vi "Replace Class Controls.vi"(8 "error in (no error)":errorcluster, 11 "Mock Class Generator In":refnum<class "Mock Class Generator.lvclass">) -> (0 "error out":errorcluster, 3 "Mock Class Generator Out":refnum<class "Mock Class Generator.lvclass">)   [LabVIEW 2020, in "Mock Class Generator.lvclass"]
uses:
  Mock Class Generator.lvclass
  Mock Class Generator.lvclass/Mock Class Generator.ctl
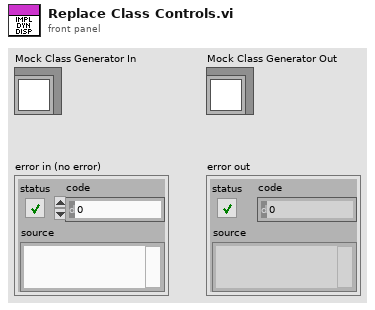
[diagram p1: front panel]
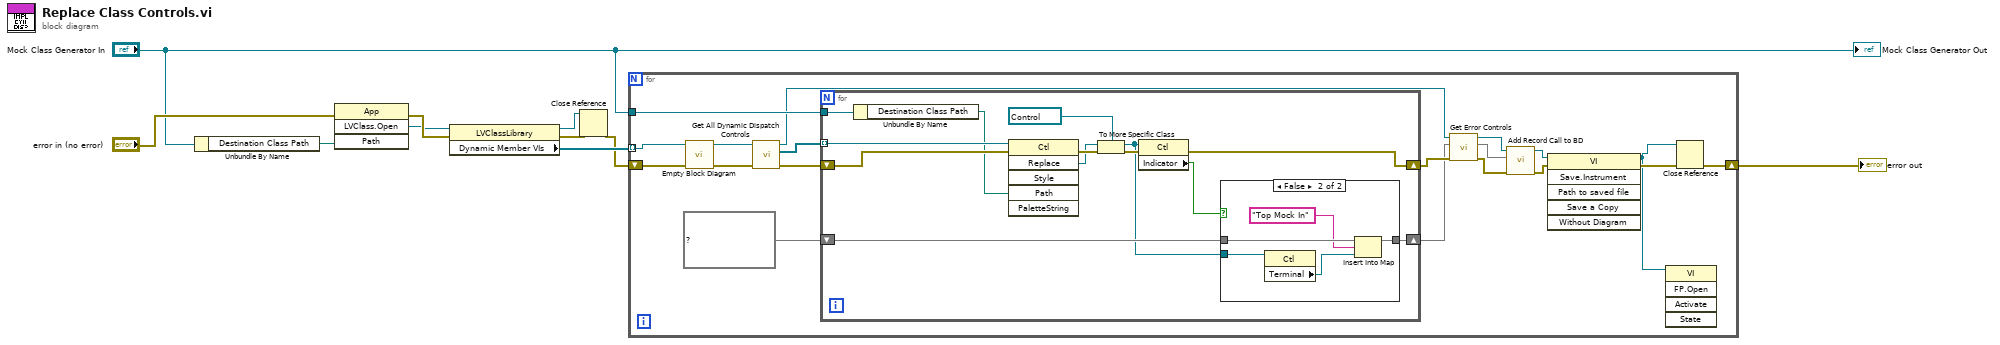
[diagram p0: block diagram]
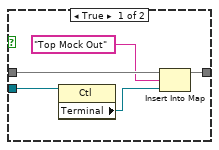
[diagram p2: hidden frame]
diagram:
  n1 = Unbundle By Name("Mock Class Generator In") -> ("Destination Class Path"=w10:path)
  n2 = invoke class="App" method="LVClass.Open"(error in="error in (no error)", "Path"=w10) -> (error out=w9:errorcluster, "LVClass.Open"=w4:refnum<vi>)  [unwired: 2 in, 2 out]
  n3 = property class="LVClassLibrary"(reference=w4, error in=w9) -> (reference out=w5:refnum<vi>, error out=w6:errorcluster, "Dynamic Member VIs"=w7:refnum<vi>[])
  n4 = Close Reference(reference=w5, error in (no error)=w6) -> (error out=w3:errorcluster)
  n5 = for {
    tunnel: w7 -> [w24] mode=indexing
    tunnel: "Mock Class Generator In" -> [w28]
    shift-right: [w25] -> w1
    shift-left: w3 -> [w21]
    n6 = call "Empty Block Diagram.vi"("error in (no error)"=w21, "VI in"=w24) -> ("error out"=w22:errorcluster, "reference out"=w23:refnum<vi>)  [unwired: 8 in]
    n7 = call "Get All Dynamic Dispatch Controls.vi"("error in (no error)"=w22, "VI in"=w23) -> ("error out"=w29:errorcluster, "Dynamic Dispatch Controls"=w27:refnum<vi>[], "reference out"=w19:refnum<vi>)  [unwired: 7 in]
    n8 = for {
      tunnel: w27 -> [w42] mode=indexing
      shift-right: [w34] -> w20
      shift-left: w29 -> [w41]
      tunnel: w28 -> [w40]
      shift-right: [w32] -> w13
      shift-left: map{string, refnum<vi>} {} ("map") -> [w33]
      n9 = Unbundle By Name(w40) -> ("Destination Class Path"=w39:path)
      n10 = invoke class="Ctl" method="Replace"(reference=w42, error in=w41, "Path"=w39) -> (error out=w38:errorcluster, "Replace"=w36:refnum<vi>)  [unwired: 3 in, 4 out]
      n11 = To More Specific Class(target class=refnum<vi> refnum ("reference out"), reference=w36, error in=w38) -> (specific class reference=w30:refnum<vi>, error out=w37:errorcluster)
      n12 = property class="Ctl"(reference=w30, error in=w37) -> (error out=w34:errorcluster, "Indicator"=w31:bool)  [unwired: 1 out]
      n13 = case shown="False" w31 {
        tunnel: w33 -> [w47 w52]
        tunnel: [w46 w51] -> w32
        tunnel: w30 -> [w44 w49]
        frame True {
          n14 = property class="Ctl"(reference=w44) -> ("Terminal"=w43:refnum<vi>)  [unwired: 1 in, 2 out]
          n15 = Insert Into Map(map in=w47, key="Top Mock Out", value=w43) -> (map out=w46:map{string, refnum<vi>})  [unwired: 2 out]
        }
        frame False {
          n16 = property class="Ctl"(reference=w49) -> ("Terminal"=w48:refnum<vi>)  [unwired: 1 in, 2 out]
          n17 = Insert Into Map(map in=w52, key="Top Mock In", value=w48) -> (map out=w51:map{string, refnum<vi>})  [unwired: 2 out]
        }
      }
    }
    n18 = call "Get Error Controls.vi"("error in (no error)"=w20, "map"=w13, "VI in"=w19) -> ("error out"=w17:errorcluster, "map out"=w12:map{string, refnum<vi>}, "reference out"=w18:refnum<vi>)  [unwired: 6 in]
    n19 = call "Add Record Call to BD.vi"("error in (no error)"=w17, "map"=w12, "VI in"=w18) -> ("error out"=w15:errorcluster, "VI out"=w16:refnum<vi>)  [unwired: 7 in]
    n20 = invoke class="VI" method="Save.Instrument"(reference=w16, error in=w15) -> (reference out=w11:refnum<vi>, error out=w26:errorcluster)  [unwired: 4 in, 4 out]
    n21 = invoke class="VI" method="FP.Open"(reference=w11) -> ()  [unwired: 4 in, 5 out]
    n22 = Close Reference(reference=w11, error in (no error)=w26) -> (error out=w25:errorcluster)
  }
  "error out" <- w1
  "Mock Class Generator Out" <- "Mock Class Generator In"
